vi "io_control_device.vi"(3 "FROM":cluster{"c2":bool, "c1":bool, "c0":bool}, 4 "TO":cluster{"c2":bool, "c1":bool, "c0":bool}, 5 "INPUT_REGS":T2, 6 "INPUT_KEYBOARD":T2) -> (0 "OUTPUT":T1, 1 "WRITE":T3, 2 "KEYBOARD_IS_ON":bool)   [LabVIEW 2013]
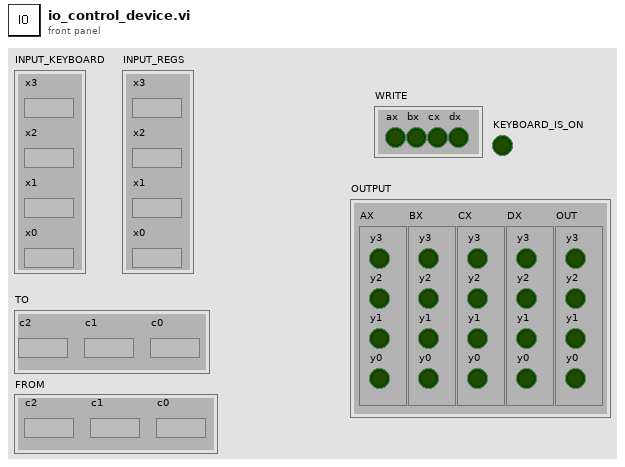
[diagram p1: front panel]
types:
  T1 = cluster{"AX":cluster{"y3":bool, "y2":bool, "y1":bool, "y0":bool}, "BX":cluster{"y3":bool, "y2":bool, "y1":bool, "y0":bool}, "CX":cluster{"y3":bool, "y2":bool, "y1":bool, "y0":bool}, "DX":cluster{"y3":bool, "y2":bool, "y1":bool, "y0":bool}, "OUT":cluster{"y3":bool, "y2":bool, "y1":bool, "y0":bool}}
  T2 = cluster{"x3":bool, "x2":bool, "x1":bool, "x0":bool}
  T3 = cluster{"ax":bool, "bx":bool, "cx":bool, "dx":bool}
  T4 = cluster{cluster{"x3":bool, "x2":bool, "x1":bool, "x0":bool}, cluster{"x3":bool, "x2":bool, "x1":bool, "x0":bool}, cluster{"x3":bool, "x2":bool, "x1":bool, "x0":bool}, cluster{"x3":bool, "x2":bool, "x1":bool, "x0":bool}, cluster{"x3":bool, "x2":bool, "x1":bool, "x0":bool}}
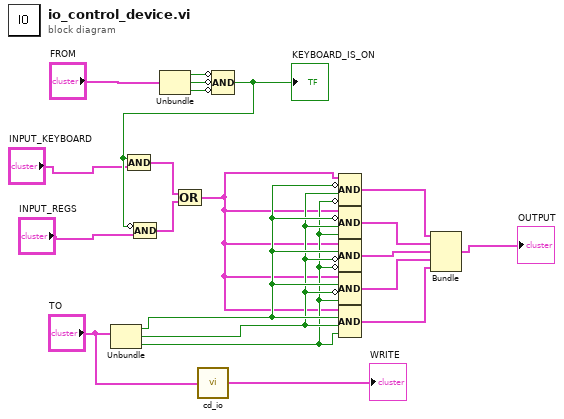
[diagram p0: block diagram]
diagram:
  n1 = Unbundle("TO") -> ("c2"=w16:bool, "c1"=w15:bool, "c0"=w14:bool)
  n2 = Unbundle("FROM") -> ("c2"=w9:bool, "c1"=w10:bool, "c0"=w11:bool)
  n3 = call "cd_io.vi"("INPUT"="TO") -> ("OUTPUT"=→"WRITE":T3)
  n4 = Compound Arithmetic op=AND(invert w9, invert w10, invert w11) -> (w7:bool)
  "KEYBOARD_IS_ON" <- w7
  n5 = Compound Arithmetic op=AND(w7, "INPUT_KEYBOARD") -> (w6:T2)
  n6 = Compound Arithmetic op=AND(invert w7, "INPUT_REGS") -> (w5:T2)
  n7 = Compound Arithmetic op=OR(w6, w5) -> (w4:T2)
  n8 = Compound Arithmetic op=AND(w4, invert w16, w15, invert w14) -> (w21:T2)
  n9 = Compound Arithmetic op=AND(w4, invert w16, w15, w14) -> (w20:T2)
  n10 = Compound Arithmetic op=AND(w4, w16, invert w15, invert w14) -> (w17:T2)
  n11 = Compound Arithmetic op=AND(w4, w16, invert w15, w14) -> (w18:T2)
  n12 = Compound Arithmetic op=AND(w4, w16, w15, w14) -> (w19:T2)
  n13 = Bundle(w21, w20, w17, w18, w19) -> (→"OUTPUT":T4)  [unwired: 1 in]
